vi "test.vi"() -> ()   [LabVIEW 2015]
panel:
  in  "Boolean 2":bool
  in  "String 2":string
  in  "Numeric 2":i32
  in  "String":string
  in  "Numeric":i32
  in  "Boolean":bool=TRUE
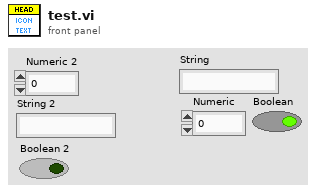
[diagram p1: front panel]
types:
  T1 = cluster{"String":string, "Numeric":i32, "Boolean":bool}
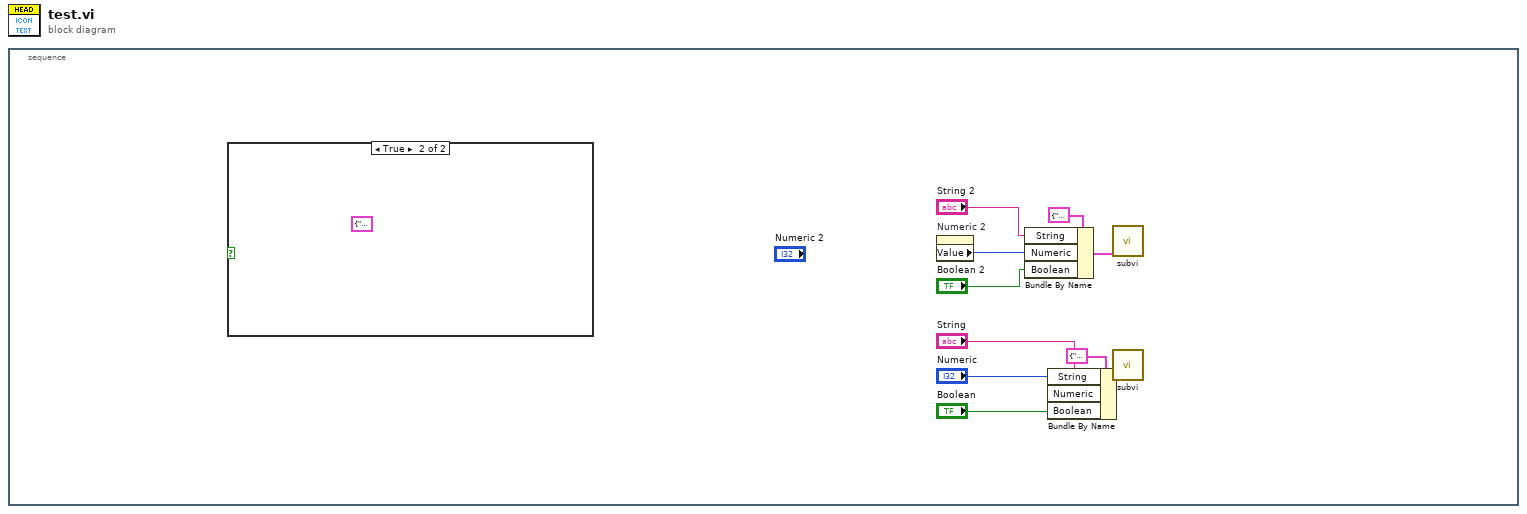
[diagram p0: block diagram]
diagram:
  n1 = stacked-sequence {
    frame #0 {
      n2 = case shown="True" {
        selector: _ -> [_ _]
        frame False {
        }
        frame True {
          (unwired) T1 {"String"="", "Numeric"=0, "Boolean"=FALSE} ("cluster in")
        }
      }
      n3 = property on="Numeric 2" class="DigNum (strict)"() -> ("Value"=w8:i32)  [unwired: 2 in, 2 out]
      n4 = Bundle By Name(cluster=T1 {"String"="", "Numeric"=0, "Boolean"=FALSE} ("cluster in"), "String"="String 2", "Numeric"=w8, "Boolean"="Boolean 2") -> (w9:T1)
      n5 = Bundle By Name(cluster=T1 {"String"="", "Numeric"=0, "Boolean"=FALSE} ("cluster in"), "String"="String", "Numeric"="Numeric", "Boolean"="Boolean") -> (w5:T1)
      n6 = call "subvi.vi"("cluster in"=w9) -> ()  [unwired: 11 in]
      n7 = call "subvi.vi"("cluster in"=w5) -> ()  [unwired: 11 in]
    }
  }
